vi "kalman_filter_1D.vi"() -> ()   [LabVIEW 2020]
panel:
  out "predict":dbl
  in  "input":dbl
  in  "system_model":cluster{"A":dbl, "H":dbl, "Q":dbl, "R":dbl}
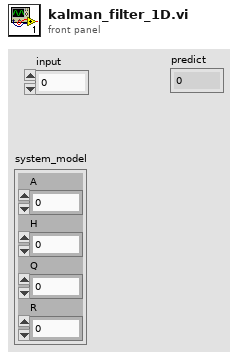
[diagram p1: front panel]
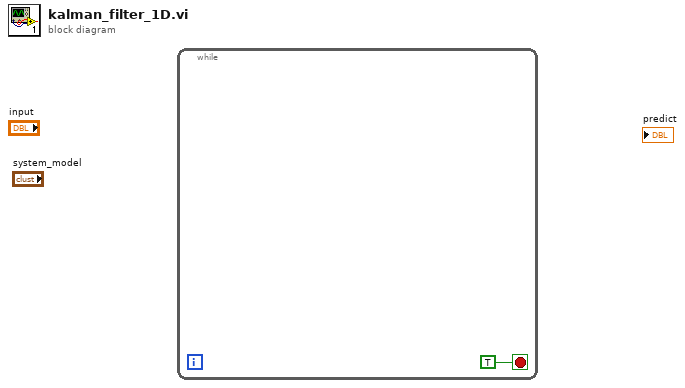
[diagram p0: block diagram]
diagram:
  n1 = while {
    stop <- TRUE stop-if-true
  }
